vi "Brushless DC Motor.vi"() -> ()   [LabVIEW 2019]
doc: "The NI ELVIS III Custom FPGA Project template acquires button data from the onboard button and displays the button value on a Boolean indicator."
uses:
  <vilib>/Platform/TimedLoop/XDataNode/timing_clust.ctl
  <vilib>/Platform/TimedLoop/XDataNode/nitl_modes.ctl
  <vilib>/Platform/TimedLoop/XDataNode/wakeup.ctl
  <vilib>/Platform/TimedLoop/XDataNode/XDataNode.xnode
  <vilib>/Platform/TimedLoop/XDataNode/XDNodeRunTimeDep.lvlib
panel:
  out "Hall Effect Sensor State":bool[](array[boolean])
  out "Error Out":errorcluster
  out "Brushless DC Motor \nSpeed (RPM)":dbl=1357.0331636287972 format="%#.0f"
  out "Brushless DC Motor Speed":dbl(graph)=1357.0331636287972
  in  "Brushless DC Motor PWM":sgl(knob) min=0 max=100 step=1 scale=0.0..100.0
  in  "Stop Button":bool
  # "Mechatronic Actuators Board"
  # "Brushless DC Motor"
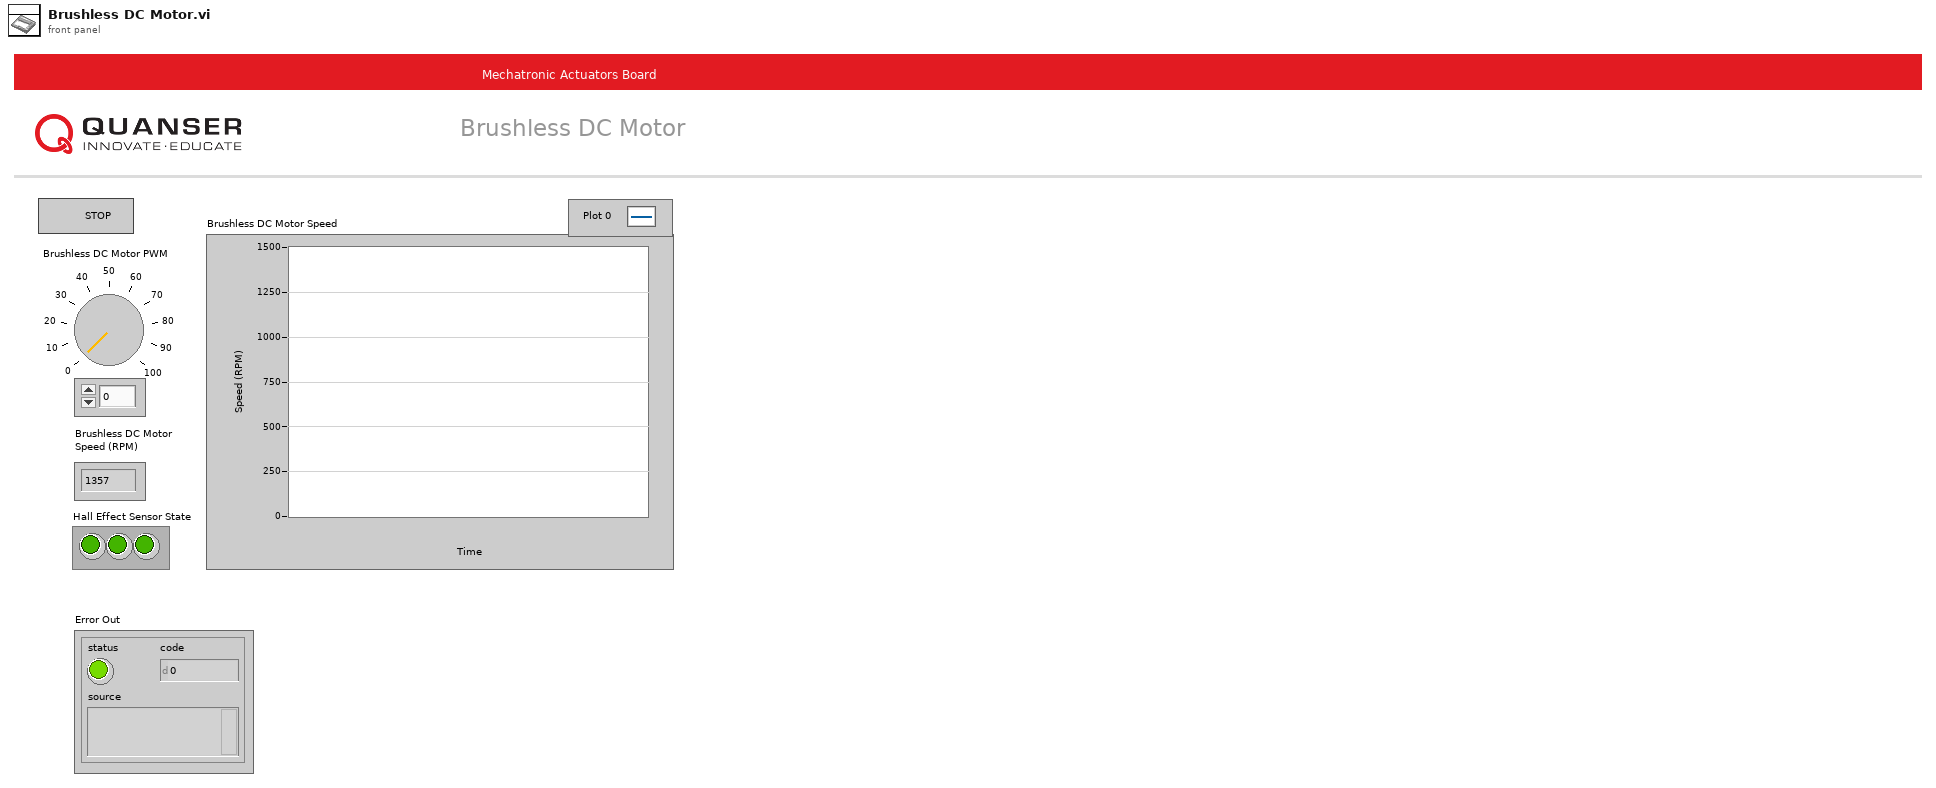
[diagram p1: front panel]
types:
  T1 = typedef "XDNodeRunTimeDep.lvlib/timing_clust.ctl" = cluster{"Expected End [f-1]":u64, "Actual End [f-1]":u64, "Finished Late? [f-1]":bool, "Expected End [i-1]":u64, "Actual End [i-1]":u64, "Finished Late? [i-1]":bool, "Expected Start [i]":u64, "Actual Start [i]":u64, "Expected Start [f]":u64, "Actual Start [f]":u64, "Source Name":string, "Structure Name":string, "Period":i64, "Deadline":i64, "Offset":i64, "Start":i64, "Priority":i32, "Timeout":i32, "Mode":T2, "Wakeup Reason":T3, "Error":errorcluster, "Source Type":string, "Secondary Source Type":string, "Global End Time":u64, "Global Start Time":u64, "Frame Duration":u64, "Iteration Duration":u64, "Assigned CPU":i32, "I/O Scan Engine Mode":u32}
  T2 = typedef "XDNodeRunTimeDep.lvlib/nitl_modes.ctl" = enum32{"No Change", "Process missed periods, maintain original phase", "Discard missed periods, maintain original phase", "Process missed periods, ignore original phase", "Discard missed periods, ignore original phase"}
  T3 = typedef "XDNodeRunTimeDep.lvlib/wakeup.ctl" = enum32{"Normal", "Aborted", "Asynchronous wakeup", "Timing source error", "Timed loop error", "Timeout"}
  T4 = typedef "Actuators IO Cluster.ctl" = cluster{"Error":errorcluster, "FPGA Ref":refnum<k20>}
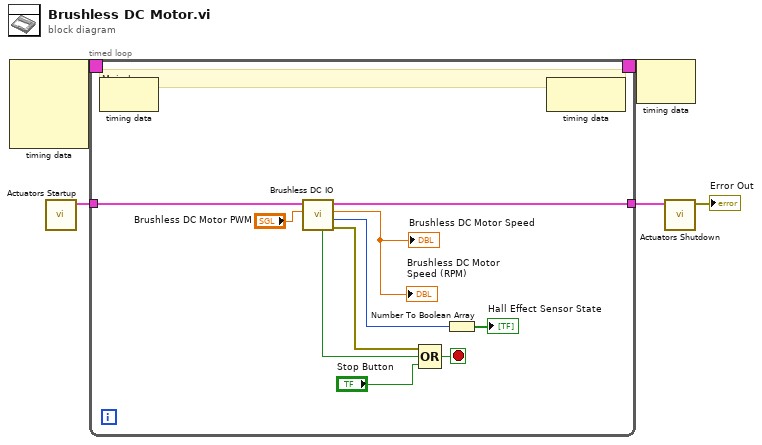
[diagram p0: block diagram]
diagram:
  n1 = node-c288() -> (w5:T1)  [unwired: 4 in]
  n2 = call "Actuators Startup.vi"() -> ("IO Cluster OUT"=w3:T4)  [unwired: 11 in]
  n3 = timed-loop {
    timing: w5 -> [_]
    timing-out: [_] -> w4
    tunnel: w3 -> [w15]
    tunnel: [w14] -> w2
    stop <- w8 stop-if-true
    # "Main Loop"
    n4 = node-c288() -> ()  [unwired: 1 in, 1 out]
    n5 = call "Brushless DC IO.vi"("Brushless DC Motor PWM"="Brushless DC Motor PWM", "IO Cluster IN"=w15) -> ("Error Out"=w9:errorcluster, "BLDC Hall Effect Sensor State"=w12:u8, "Brushless DC Motor Speed (RPM)"=→"Brushless DC Motor Speed" →"Brushless DC Motor \nSpeed (RPM)":dbl, "IO Cluster OUT"=w14:T4, "Hall Effect Sensor Error"=w7:bool)  [unwired: 5 in]
    n6 = Compound Arithmetic op=OR(w9, w7, "Stop Button") -> (w8:bool)
    n7 = Number To Boolean Array(number=w12) -> (Boolean array=→"Hall Effect Sensor State":bool[])
    n8 = node-c288() -> ()  [unwired: 1 in, 1 out]
  }
  n9 = node-c288(w4) -> ()  [unwired: 1 out]
  n10 = call "Actuators Shutdown.vi"("IO Cluster IN"=w2) -> ("Error Out"=→"Error Out":errorcluster)  [unwired: 10 in]
